vi "SimplePowMap.vi"(8 "Low":dbl, 9 "High":dbl, 11 "LineOut":dbl[](array[numeric])) -> (3 "Mapped":dbl[](array[numeric]))   [LabVIEW 2014]
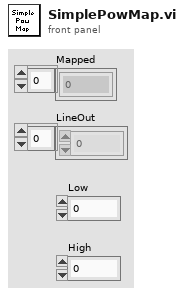
[diagram p1: front panel]
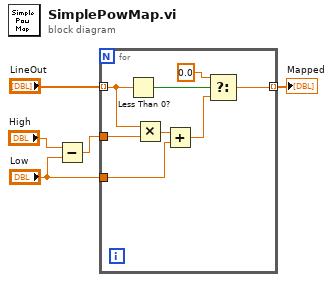
[diagram p0: block diagram]
diagram:
  n1 = Subtract(x="High", y="Low") -> (x-y=w3:dbl)
  n2 = for {
    tunnel: "LineOut" -> [w11] mode=indexing
    tunnel: w3 -> [w10]
    tunnel: "Low" -> [w8]
    tunnel: [w6] -> w1 mode=indexing
    n3 = Less Than 0?(x=w11) -> (x < 0?=w13:bool)
    n4 = Multiply(x=w11, y=w10) -> (x*y=w9:dbl)
    n5 = Add(x=w9, y=w8) -> (x+y=w7:dbl)
    n6 = Select(t=0.0, s=w13, f=w7) -> (s? t:f=w6:dbl)
  }
  "Mapped" <- w1
